vi "Test Class Decompose Recompose.vi"() -> ()   [LabVIEW 2026, in "VILab.lvlib"]
uses:
  VILab.lvlib
  SubVIs/Decompose VI (Refnum).vi
  <userlib>/_OpenG.lib/array/array.llb/Filter 1D Array with Scalar (Boolean)__ogtk.vi
  SubVIs/Classes/Attribute/Attribute.lvclass
  <userlib>/_OpenG.lib/array/array.llb/openg_array.lvlib
panel:
  out "filtered item indices 2":i32[](array[numeric])
  out "filtered item indices":i32[](array[numeric])
  out "Block Diagram XML":string
  out "Front Panel XML":string
  out "Rebuilt BD XML":string
  out "Rebuilt FP XML":string
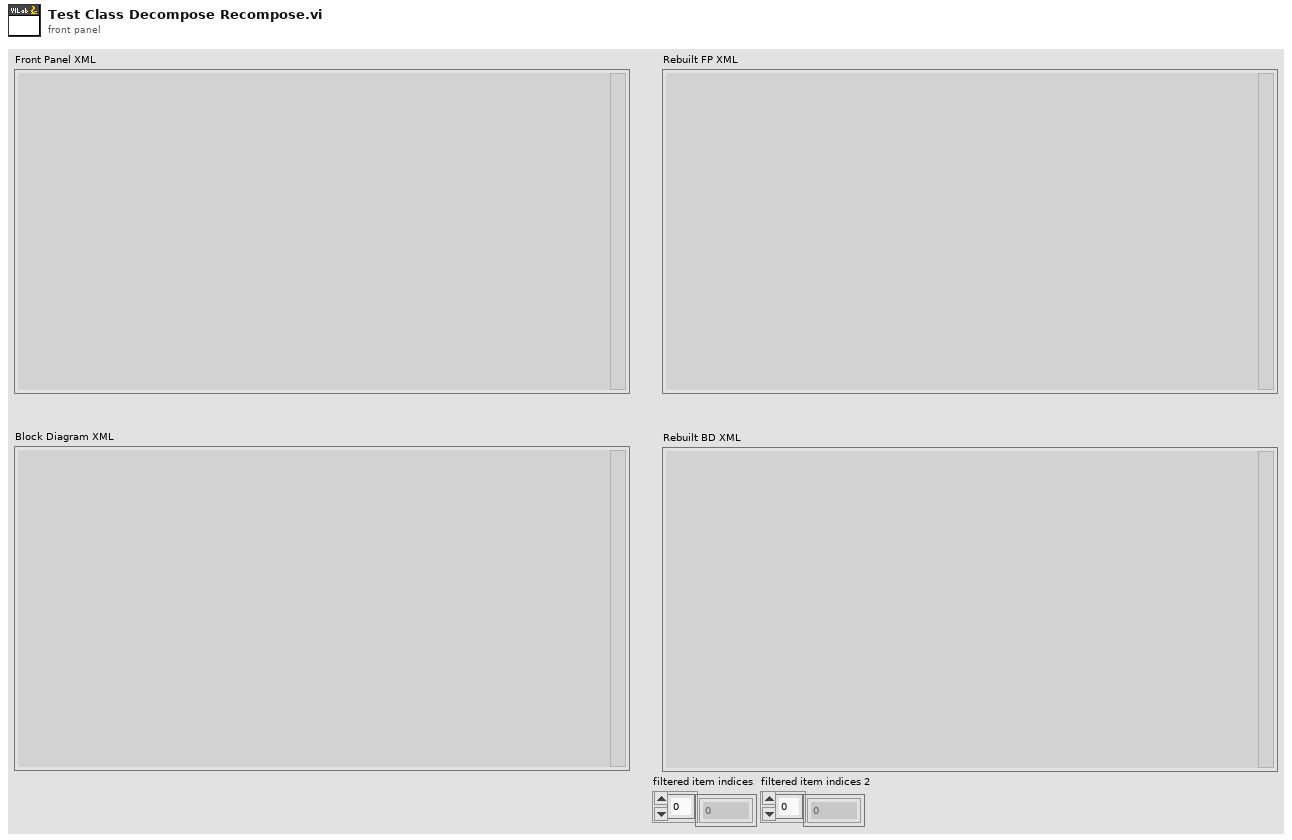
[diagram p1: front panel]
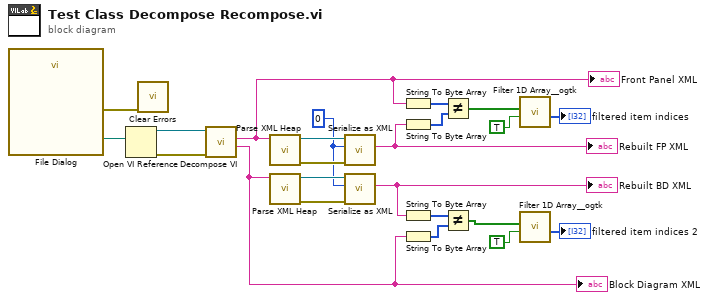
[diagram p0: block diagram]
diagram:
  w15 = 0 ("Nesting Level")
  n1 = call "File Dialog"() -> ("selected path"=w17:path, "error out"=w16:errorcluster)  [unwired: 12 in, 2 out]
  n2 = Open VI Reference(vi path=w17) -> (vi reference=w23:refnum<vi>, error out=w18:errorcluster)  [unwired: 5 in]
  n3 = call <vilib>:"Clear Errors.vi"("error in (no error)"=w16) -> ()  [unwired: 5 in, 2 out]
  n4 = call-poly "Decompose VI.vi"("error in (no error)"=w18, "VI Ref"=w23) -> ("Block Diagram XML"=w11:string, "Front Panel XML"=w14:string)  [unwired: 5 in, 3 out]
  "Front Panel XML" <- w14
  "Block Diagram XML" <- w11
  n5 = call "Parse XML Heap.vi"("XML"=w14) -> ("error out"=w20:errorcluster, "Root Element"=w22:refnum<class "Attribute.lvclass">)  [unwired: 9 in]
  n6 = call "Parse XML Heap.vi"("XML"=w11) -> ("error out"=w19:errorcluster, "Root Element"=w21:refnum<class "Attribute.lvclass">)  [unwired: 9 in]
  n7 = call-dynamic "Serialize as XML.vi"("error in (no error)"=w20, "Nesting Level"=w15, "Attribute in"=w22) -> ("XML Fragment"=w13:string)  [unwired: 6 in, 2 out]
  "Rebuilt FP XML" <- w13
  n8 = call-dynamic "Serialize as XML.vi"("error in (no error)"=w19, "Nesting Level"=w15, "Attribute in"=w21) -> ("XML Fragment"=w12:string)  [unwired: 6 in, 2 out]
  "Rebuilt BD XML" <- w12
  n9 = String To Byte Array(string=w14) -> (unsigned byte array=w10:u8[])
  n10 = String To Byte Array(string=w13) -> (unsigned byte array=w9:u8[])
  n11 = String To Byte Array(string=w12) -> (unsigned byte array=w8:u8[])
  n12 = String To Byte Array(string=w11) -> (unsigned byte array=w7:u8[])
  n13 = Not Equal?(x=w10, y=w9) -> (x != y?=w6:bool[])
  n14 = Not Equal?(x=w8, y=w7) -> (x != y?=w1:bool[])
  n15 = call-poly <userlib>:"Filter 1D Array__ogtk.vi"("items to filter"=TRUE, "array"=w6) -> ("filtered item indices"=→"filtered item indices":i32[])  [unwired: 4 in, 1 out]
  n16 = call-poly <userlib>:"Filter 1D Array__ogtk.vi"("items to filter"=TRUE, "array"=w1) -> ("filtered item indices"=→"filtered item indices 2":i32[])  [unwired: 4 in, 1 out]
